vi "pcap dump open.vi"(8 "error in":errorcluster, 10 "capture file path":path=path "/home/lvuser/test.pcap", 11 "pcap_t in":u64) -> (0 "error out":errorcluster, 2 "pcap_dumper_t":u64, 3 "pcap_t out":u64)   [LabVIEW 2020, in "libpcaplv.lvlib"]
uses:
  libpcaplv.lvlib
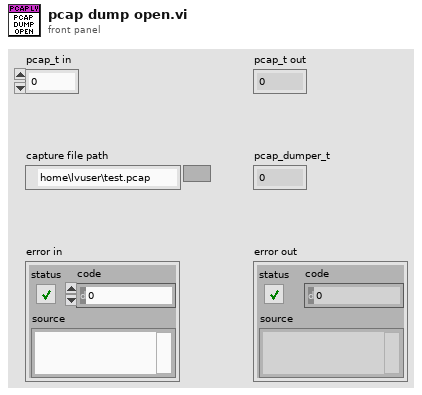
[diagram p1: front panel]
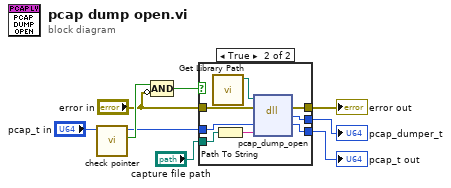
[diagram p0: block diagram]
diagram:
  n1 = call "check pointer.vi"("pointer in"="pcap_t in") -> ("ok"=w8:bool, "pointer out"=w6:u64)  [unwired: 9 in]
  n2 = Compound Arithmetic op=AND(w8, invert "error in") -> (w5:bool)
  n3 = case shown="True" w5 {
    tunnel: [w10 w19] -> w9
    tunnel: w6 -> [w11 w17]
    tunnel: "error in" -> [w10 w18]
    tunnel: "capture file path" -> [_ w16]
    tunnel: [w11 w14] -> w2
    tunnel: [_ w13] -> w1
    frame False {
    }
    frame True {
      n4 = call "Get Library Path.vi"() -> ("library path"=w12:path)  [unwired: 11 in]
      n5 = Path To String(path=w16) -> (string=w15:string)
      n6 = dll-call lib="libpcap.*" fn="pcap_dump_open"(path in=w12, error in=w18, "pcap_t"=w17, "fname"=w15) -> (error out=w19:errorcluster, "pcap_dumper_t"=w13:u64, "pcap_t"=w14:u64)  [unwired: 2 in, 1 out]
    }
  }
  "pcap_t out" <- w2
  "error out" <- w9
  "pcap_dumper_t" <- w1
